vi "StartCalibration.vi"(4 "error in":errorcluster, 7 "Queues Cluster":T1) -> (0 "error out":errorcluster, 3 "Started?":bool)   [LabVIEW 2017]
uses:
  SubVIQueues.ctl
  AODControl/MessageQueue/QueueOperations/All Message Queues.ctl
  AODControl/MessageQueue/QueueOperations/Message Cluster.ctl
  MessageQueue/QueueOperations/Enqueue Message (Single).vi
  MessageQueue/MessageQueue.lvlib
  AODControl/MessageQueue/MessageQueue.lvlib
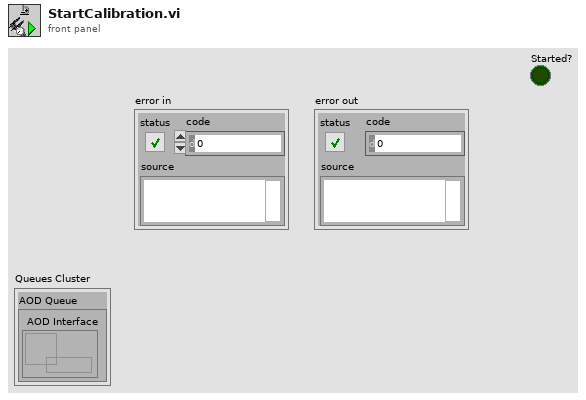
[diagram p1: front panel]
types:
  T1 = typedef "SubVIQueues.ctl" = cluster{"AOD Queue":T2}
  T2 = typedef "AODControl.lvlib/MessageQueue.lvlib/All Message Queues.ctl" = cluster{" AOD Interface":refnum<queue>}
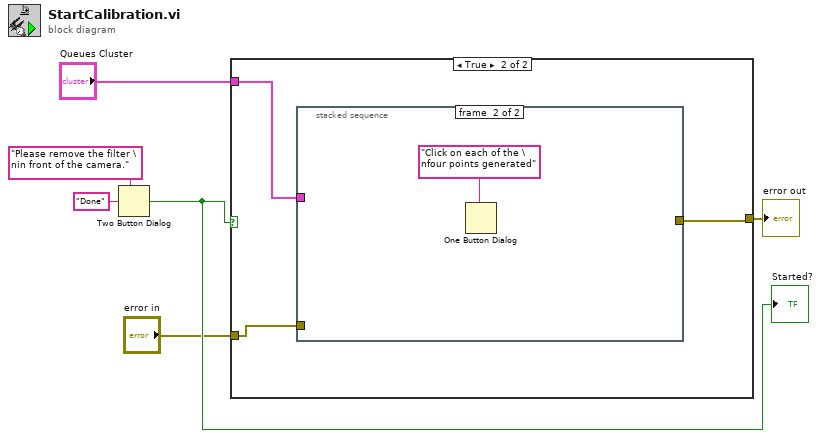
[diagram p0: block diagram]
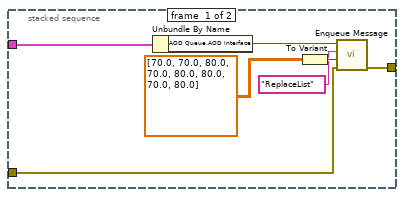
[diagram p3: hidden frame]
diagram:
  n1 = Two Button Dialog(message="Please remove the filter \nin front of the camera.", 2:"Done" ("T button name (\"OK\")")) -> (T button?=w5:bool)  [unwired: 1 in]
  "Started?" <- w5
  n2 = case shown="True" w5 {
    tunnel: "Queues Cluster" -> [_ w10]
    tunnel: [w7 w9] -> w2
    tunnel: "error in" -> [w7 w8]
    frame False {
    }
    frame True {
      n3 = stacked-sequence {
        tunnel: w10 -> [w13 _]
        tunnel: [w12 _] -> w9
        tunnel: w8 -> [w11 _]
        frame #0 {
          n4 = Unbundle By Name(w13) -> ("AOD Queue.AOD Interface"=w17:refnum<queue>)
          n5 = To Variant(anything=dbl[][] [[70.0, 70.0], [80.0, 70.0], [80.0, 80.0], [70.0, 80.0]] ("Array")) -> (Variant=w16:variant)
          n6 = call-poly "Enqueue Message.vi"("error in (no error)"=w11, "Message Data"=w16, "Message"="ReplaceList", "Message Queue"=w17) -> ("error out"=w12:errorcluster)  [unwired: 6 in, 1 out]
        }
        frame #1 {
          n7 = One Button Dialog(message="Click on each of the \nfour points generated") -> ()  [unwired: 1 in, 1 out]
        }
      }
    }
  }
  "error out" <- w2
